vi "XY Galvo With Homography.vi"(0 "Exposure (ms)":dbl=10.0 format="%0.2p", 1 "Underscan /ms":dbl, 2 "Camera Delay /ms":dbl, 4 "Samples /Millisecond":dbl=10.0 format="%0.2p", 5 "Relax (ms)":dbl=10.0 format="%0.2p", 18 "Piezo Position (um)":dbl) -> (14 "Scan Mirror Signal":dbl[](graph), 15 "Piezo Signal":dbl[](graph), 16 "Camera Signal":dbl[](graph), 17 "Laser Signal":dbl[](graph), 19 "Z Mirror Signal":dbl[](graph))   [LabVIEW 2015]
uses:
  GlobalVariables.vi
  <vilib>/Analysis/NI_AALBase.lvlib
panel:
  out "Time Taken (ms)":dbl
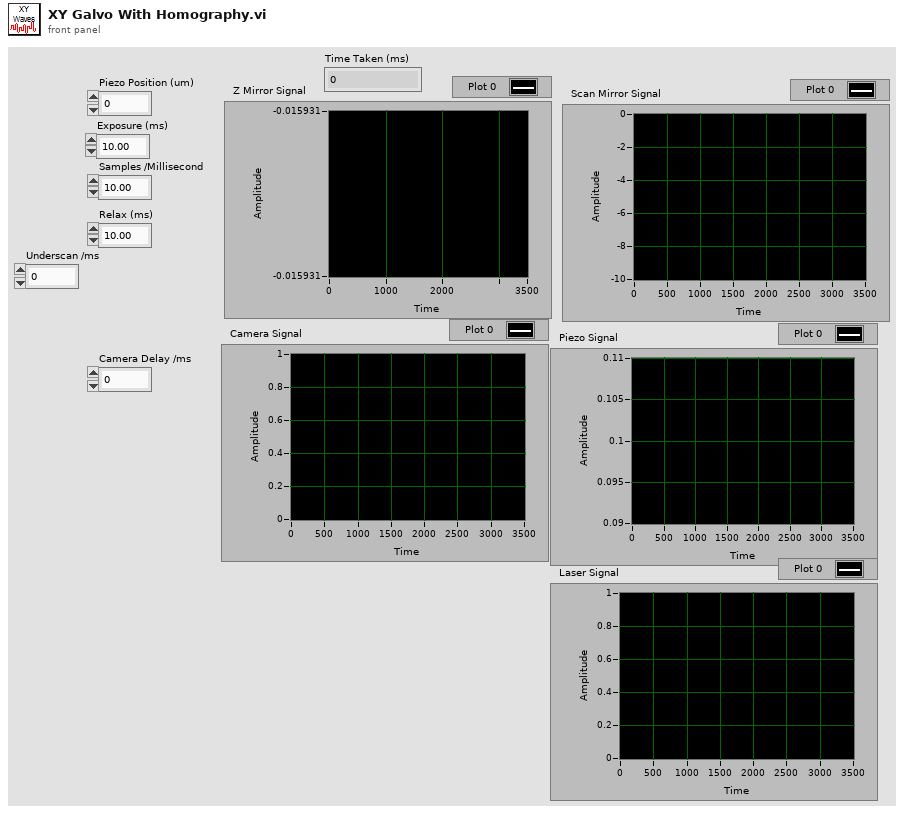
[diagram p1: front panel]
types:
  T1 = cluster{"Top Left":dbl[], "Top Right":dbl[], "Bottom Left":dbl[], "Bottom Right":dbl[]}
  T2 = typedef "NI_Matrix.lvlib/RealMatrix.ctl" = dbl[][]
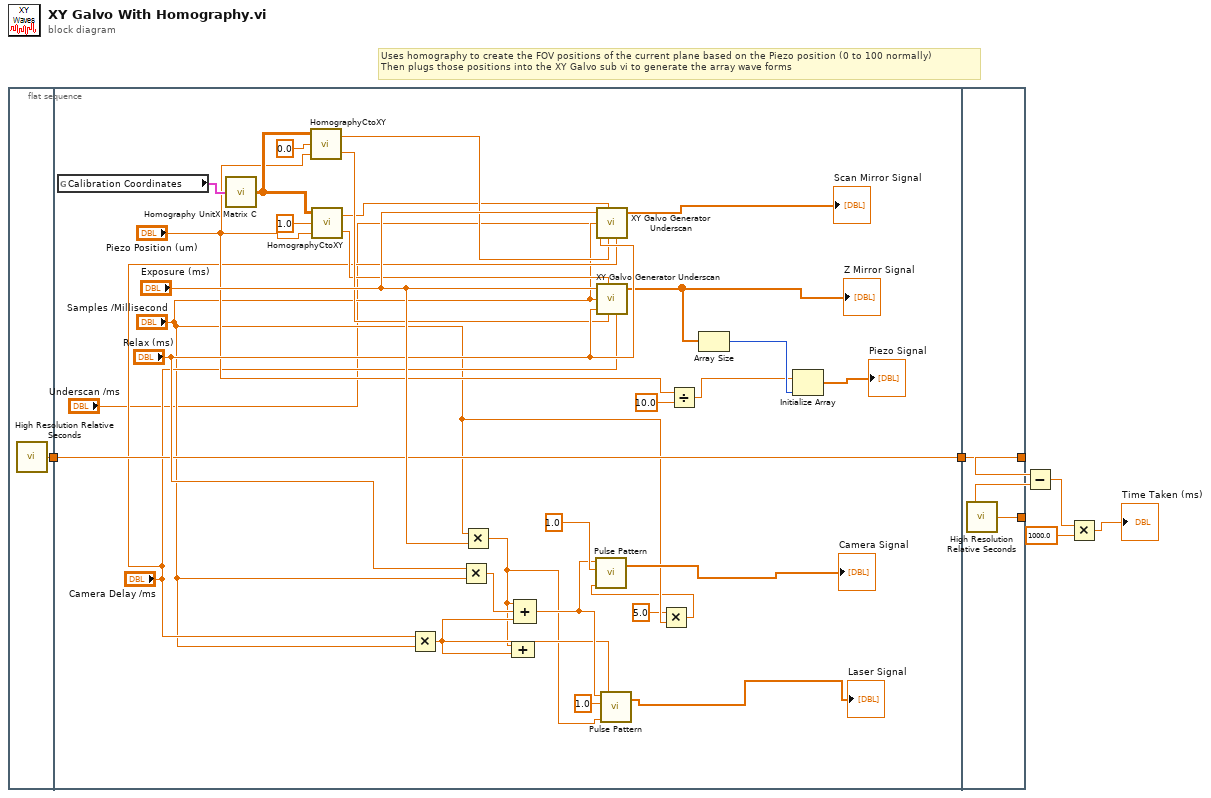
[diagram p0: block diagram]
diagram:
  # "Uses homography to create the FOV positions of the current plane based on the Piezo position (0 to 100 normally)\nThen plugs those positions into the XY Galvo sub vi to generate the array wave forms"
  n1 = flat-sequence {
    tunnel: [w8] -> w6
    tunnel: [w28] -> w7
    tunnel: w6 -> [w28]
    tunnel: w7 -> [w41]
    tunnel: [w41] -> w5
    tunnel: [w40] -> w4
    frame #0 {
      n2 = call <vilib>:"High Resolution Relative Seconds.vi"() -> ("relative seconds"=w8:dbl)
    }
    frame #1 {
      n3 = global read "GlobalVariables.vi" "Calibration Coordinates"() -> (w36:T1)
      n4 = call "Homography UnitX Matrix C.vi"("input cluster"=w36) -> ("C"=w33:T2)
      n5 = call "HomographyCtoXY.vi"("Y"="Piezo Position (um)", "X"=0.0, "C"=w33) -> ("Y"=w32:dbl, "X"=w30:dbl)
      n6 = call "HomographyCtoXY.vi"("Y"="Piezo Position (um)", "X"=1.0, "C"=w33) -> ("Y"=w31:dbl, "X"=w29:dbl)
      n7 = Multiply(x="Camera Delay /ms", y="Samples /Millisecond") -> (x*y=w16:dbl)
      n8 = Multiply(x="Relax (ms)", y="Samples /Millisecond") -> (x*y=w20:dbl)
      n9 = Multiply(x="Samples /Millisecond", y="Exposure (ms)") -> (x*y=w15:dbl)
      n10 = Compound Arithmetic op=ADD(w15, w16) -> ()  [unwired: 1 out]
      n11 = Compound Arithmetic op=ADD(w15, w20, w16) -> (w18:dbl)
      n12 = call "XY Galvo Generator Underscan.vi"("Exposure /ms"="Exposure (ms)", "FOV max / V"=w29, "Samples per ms"="Samples /Millisecond", "Relax /ms"="Relax (ms)", "FOV min/ V"=w30, "Underscan /ms"="Underscan /ms", "Delay /ms"="Camera Delay /ms") -> ("Signal"=→"Scan Mirror Signal":dbl[])  [unwired: 2 in]
      n13 = call "XY Galvo Generator Underscan.vi"("Exposure /ms"="Exposure (ms)", "FOV max / V"=w31, "Samples per ms"="Samples /Millisecond", "Relax /ms"="Relax (ms)", "FOV min/ V"=w32, "Delay /ms"="Camera Delay /ms") -> ("Signal"=w27:dbl[])  [unwired: 3 in]
      "Z Mirror Signal" <- w27
      n14 = call <vilib>:"Pulse Pattern.vi"("width"=w15, "delay"=w16, "amplitude"=1.0, "samples"=w18) -> ("Pulse Pattern"=→"Laser Signal":dbl[])  [unwired: 1 out]
      n15 = Multiply(x=5.0, y="Samples /Millisecond") -> (x*y=w10:dbl)
      n16 = call <vilib>:"Pulse Pattern.vi"("width"=w10, "amplitude"=1.0, "samples"=w18) -> ("Pulse Pattern"=→"Camera Signal":dbl[])  [unwired: 1 in, 1 out]
      n17 = Divide(x="Piezo Position (um)", y=10.0) -> (x/y=w23:dbl)
      n18 = Array Size(array=w27) -> (size(s)=w26:i32)
      n19 = Initialize Array(w23, w26) -> (→"Piezo Signal":dbl[])
    }
    frame #2 {
      n20 = call <vilib>:"High Resolution Relative Seconds.vi"() -> ("relative seconds"=w40:dbl)
    }
  }
  n21 = Subtract(x=w5, y=w4) -> (x-y=w3:dbl)
  n22 = Multiply(x=w3, y=1000.0) -> (x*y=→"Time Taken (ms)":dbl)
